vi "SCT Launch SubVIs.vi"(5 "names":string[](array[string]), 7 "var type paths":path[](array[path]), 9 "localized names":string[](array[string]), 10 "broadcast user event":T4, 11 "Project Refnum":refnum<vi>) -> (1 "Localized Names Out":string[](array[string]), 2 "Feature Pack Info":T3(array[cluster]), 3 "Project Refnum out":refnum<vi>)   [LabVIEW 2016]
uses:
  <resource>/dialog/variable/SCT Broadcast User Event.ctl
  <resource>/dialog/variable/SCT Broadcast.ctl
  <resource>/dialog/variable/SCT Message User Event.ctl
  <resource>/dialog/variable/SCT Message.ctl
  <vilib>/variable/Type Descriptor.ctl
  <resource>/dialog/variable/SCT Attributes.ctl
  <resource>/dialog/variable/SCT Attributes Event.ctl
  <vilib>/Utility/error.llb/DialogType.ctl
  <resource>/dialog/variable/SCT Localization Strings.vi
  <vilib>/variable/NI_Variable.lvlib
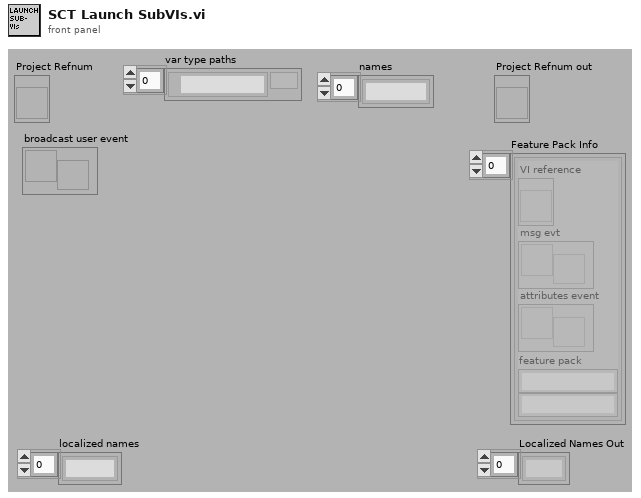
[diagram p1: front panel]
types:
  T1 = typedef "SCT Message User Event.ctl" = refnum<user-event>
  T2 = typedef "SCT Attributes Event.ctl" = refnum<user-event>
  T3 = cluster{"VI reference":refnum<vi>, "msg evt":T1, "attributes event":T2, "feature pack":string, string}[]
  T4 = typedef "SCT Broadcast User Event.ctl" = refnum<user-event>
  T5 = cluster{"VI reference":refnum<vi>, "msg evt":T1, "attributes event":T2, "feature pack":string, string}
  T6 = typedef "DialogType.ctl" = u16
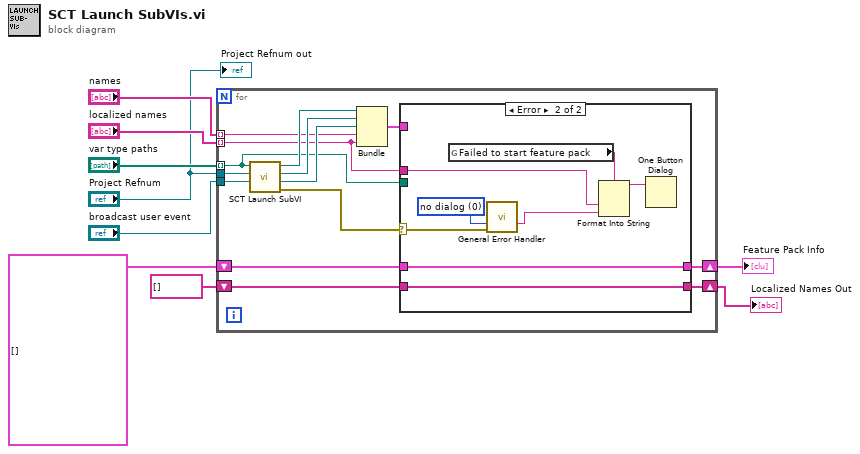
[diagram p0: block diagram]
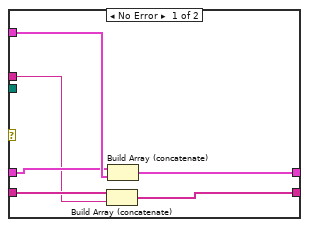
[diagram p2: hidden frame]
diagram:
  n1 = for {
    tunnel: "names" -> [w20] mode=indexing
    tunnel: "var type paths" -> [w13] mode=indexing
    tunnel: "Project Refnum" -> [w19]
    tunnel: "broadcast user event" -> [w18]
    tunnel: "localized names" -> [w12] mode=indexing
    shift-right: [w15] -> w6
    shift-left: T3 [] -> [w16]
    shift-right: [w10] -> w2
    shift-left: string[] [] -> [w11]
    n2 = call <resource>:"SCT Launch SubVI.vi"("broadcast user event"=w18, "Project Refnum"=w19, "subVI path"=w13) -> ("error out"=w17:errorcluster, "attributes event"=w21:T2, "msg evt"=w22:T1, "VI reference"=w23:refnum<vi>)  [unwired: 5 in]
    n3 = Bundle("VI reference"=w23, "msg evt"=w22, "attributes event"=w21, "feature pack"=w20, w12) -> (w14:T5)  [unwired: 1 in]
    n4 = case shown="Error" w17 {
      selector: w17 -> [_ w35]
      tunnel: [w29 w37] -> w15
      tunnel: w16 -> [w27 w37]
      tunnel: w14 -> [w28 _]
      tunnel: w12 -> [w24 w32]
      tunnel: w13 -> [_ _]
      tunnel: w11 -> [w26 w31]
      tunnel: [w25 w31] -> w10
      frame No Error {
        n5 = Build Array (concatenate)(w26, w24) -> (w25:string[])
        n6 = Build Array (concatenate)(w27, w28) -> (w29:T3)
      }
      frame Error {
        w34 = T6 0 items=["no dialog", "OK message", "continue or stop message", "OK message + warnings", "continue/stop + warnings"] ("type of dialog (OK msg:1)")
        n7 = global read "SCT Localization Strings.vi" "Failed to start feature pack"() -> (w36:string)
        n8 = call <vilib>:"General Error Handler.vi"("type of dialog (OK msg:1)"=w34, "error in (no error)"=w35) -> ("message"=w33:string)  [unwired: 9 in, 4 out]
        n9 = Format Into String(format string=w36, w32, w33) -> (resulting string=w30:string)  [unwired: 2 in, 1 out]
        n10 = One Button Dialog(message=w30) -> ()  [unwired: 1 in, 1 out]
      }
    }
  }
  "Feature Pack Info" <- w6
  "Localized Names Out" <- w2
  "Project Refnum out" <- "Project Refnum"
